vi "Standby Power Header.vi"(8 "Error In":errorcluster, 11 "Array":string[](array[string])) -> (0 "Error Out":errorcluster, 3 "Header File":string[][](array[string])=[["Instrument", "YOKOGAWA,WT332,C2QB17128V,F1.03\n"], ["Instr Driver Revision", "1.0 F1.03"], ["Start Time", "1.0"], ["Voltage Range", "6/1/2015 11:50 AM"], ["Current Range", "Auto"], ["Update Rate", "Auto"], ["Standard", "0.250"], ["Algorithm", "IEC62301 Ed.2(Auto)"], ["Stop Factor", "Linear Regression"], ["Valid Period", ""], ["Start Total Harmonic Distortion Uthd 1", "0.065"], ["Start Total Harmonic Distortion Uthd 2", ""], ["End Total Harmonic Distortion Uthd 1", ""], ["End Total Harmonic Distortion Uthd 2", ""], ["Max Power (Watts)", ""], ["Power Variation (%)", ""], ["", ""]])   [LabVIEW 2018]
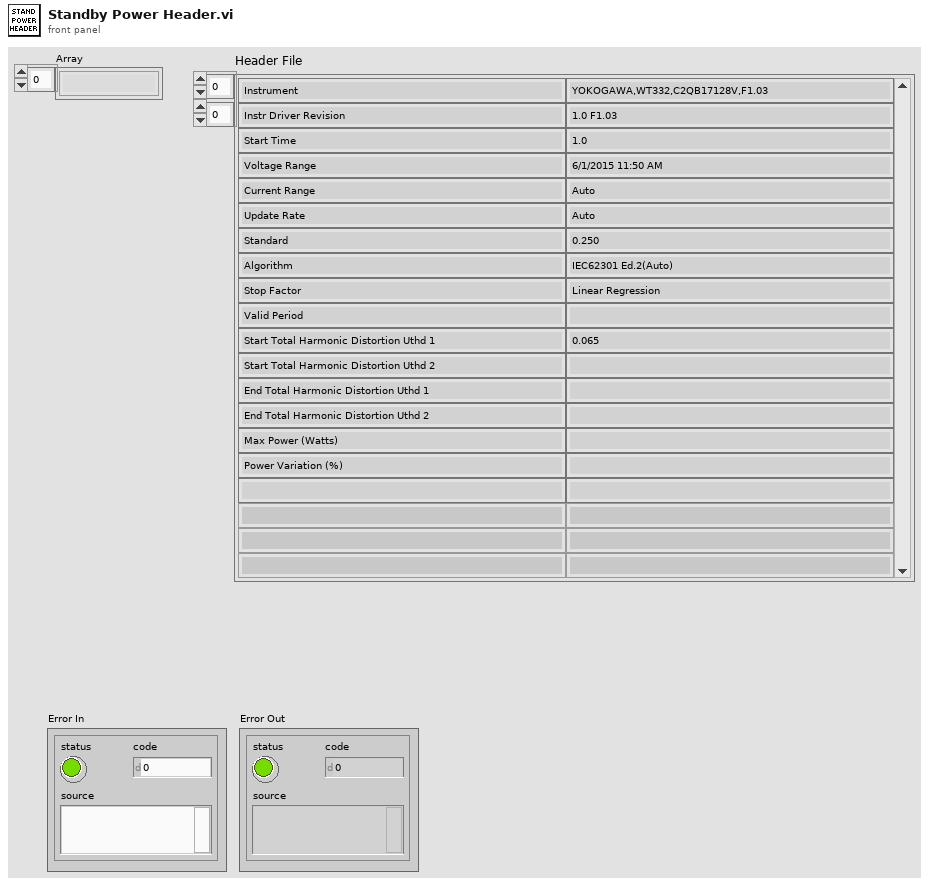
[diagram p1: front panel]
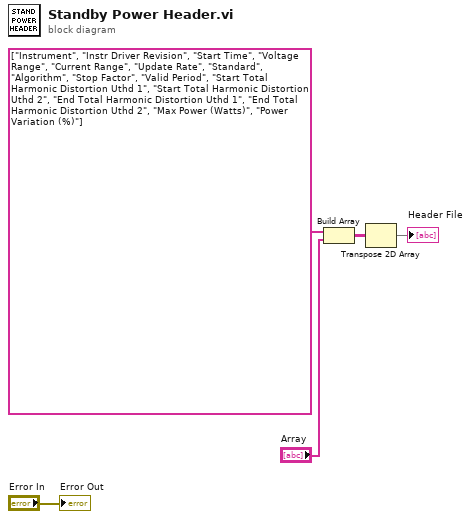
[diagram p0: block diagram]
diagram:
  n1 = Build Array(string[] ["Instrument", "Instr Driver Revision", "Start Time", "Voltage Range", "Current Range", "Update Rate", "Standard", "Algorithm", "Stop Factor", "Valid Period", "Start Total Harmonic Distortion Uthd 1", "Start Total Harmonic Distortion Uthd 2", "End Total Harmonic Distortion Uthd 1", "End Total Harmonic Distortion Uthd 2", "Max Power (Watts)", "Power Variation (%)"], "Array") -> (w3:string[][])
  n2 = Transpose 2D Array(2D array=w3) -> (transposed array=→"Header File":string[][])
  "Error Out" <- "Error In"
